vi "Error Read.vi"(8 "error in":errorcluster, 11 "Cycler in":refnum<class "Cycler.lvclass">) -> (0 "error out":errorcluster, 1 "Changed or First Call?":bool, 2 "Error ACT":bool, 3 "Cycler out":refnum<class "Cycler.lvclass">)   [LabVIEW 2023, in "Cycler.lvclass"]
uses:
  Cycler.lvclass
  Cycler.lvclass/Cycler.ctl
  Low Level Capabilities/Error/Error.lvclass
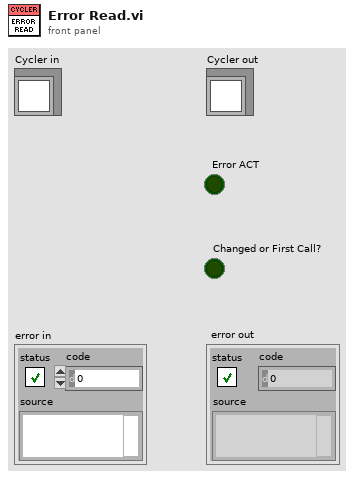
[diagram p1: front panel]
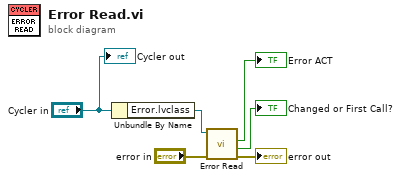
[diagram p0: block diagram]
diagram:
  n1 = Unbundle By Name("Cycler in") -> ("Error.lvclass"=w6:refnum<class "Error.lvclass">)
  n2 = call-dynamic "Error Read.vi"("error in"="error in", "Error in"=w6) -> ("error out"=→"error out":errorcluster, "Changed or First Call?"=→"Changed or First Call?":bool, "Error ACT"=→"Error ACT":bool)  [unwired: 6 in, 1 out]
  "Cycler out" <- "Cycler in"
